vi "enableSCurve.vi"(0 "MultiAxisController in":refnum<class "_MultiAxisController.lvclass">, 2 "axis":T1, 5 "error in (no error)":errorcluster) -> (14 "MultiAxisController out":refnum<class "_MultiAxisController.lvclass">, 17 "success?":bool, 18 "response":string, 19 "error out":errorcluster)   [LabVIEW 2020, in "classes.lvlib" / "_MultiAxisController.lvclass"]
doc: "Enable S Curve for a typical multi-axis controller\n\nProduced By:\n\n<B>Kod Integrations, LLC</B>\n4835 Marianne Drive\nMount Airy, MD 21771\nhttp://www.kodintegrations.com\nemail: info@kodintegrations.com\nphone: (240) 687-1288"
uses:
  _MultiAxisController.lvclass
  C:/GEECS/Developers Version/source/Device Drivers/Newmark-NSC-A/Arcus Driver 3.0.0/ArcusUsbComm/classes/Controller/_Controller.lvclass
  common/controls/axis.ctl
  Controller/_Controller.lvclass
  libraries/common.lvlib
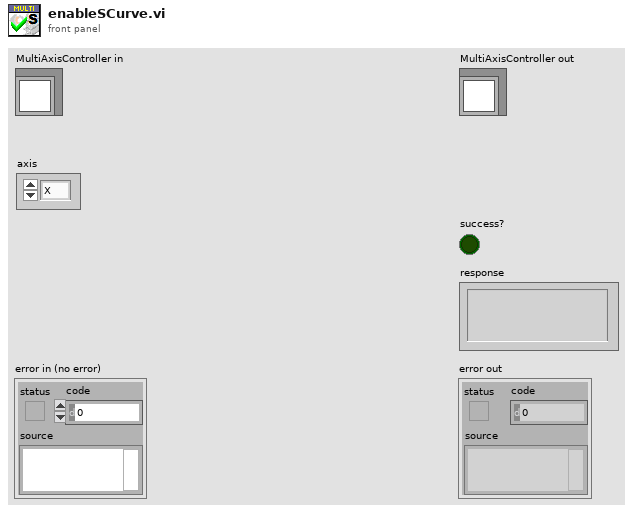
[diagram p1: front panel]
types:
  T1 = typedef "common.lvlib/axis.ctl" = enum16{"X", "Y", "Z", "U"}
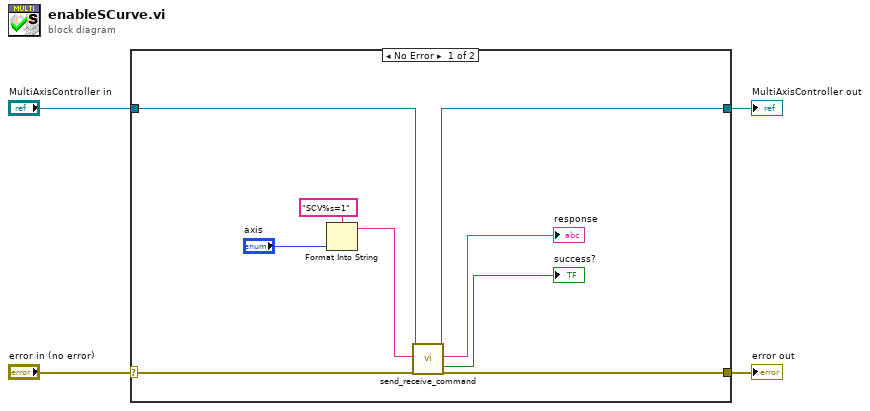
[diagram p0: block diagram]
diagram:
  n1 = case shown="No Error" "error in (no error)" {
    selector: "error in (no error)" -> [w8 w15]
    tunnel: [w7 w15] -> w3
    tunnel: [w5 w14] -> w1
    tunnel: "MultiAxisController in" -> [w6 w14]
    frame No Error {
      n2 = Format Into String(format string="SCV%s=1", "axis") -> (resulting string=w11:string)  [unwired: 2 in, 1 out]
      n3 = call "send_receive_command.vi"("reference (in)"=w6, "ASCII Command (in)"=w11, "error in (no error)"=w8) -> ("reference (out)"=w5:refnum<class "_MultiAxisController.lvclass">, "response (out)"=→"response":string, "success?"=→"success?":bool, "error out"=w7:errorcluster)  [unwired: 12 in, 1 out]
    }
    frame Error {
    }
  }
  "error out" <- w3
  "MultiAxisController out" <- w1
